vi "sub_calAzimuth.vi"(10 "Index (data block)":i32, 11 "Byte Array":u8[](array[numeric]) format="%x") -> (3 "Azimuth (degree)":dbl format="%#.6f")   [LabVIEW 2020]
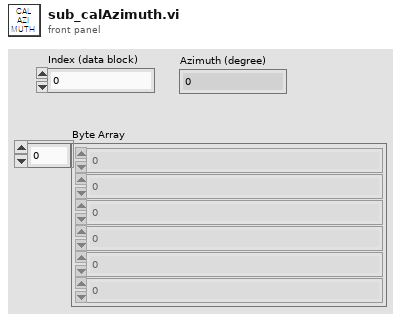
[diagram p1: front panel]
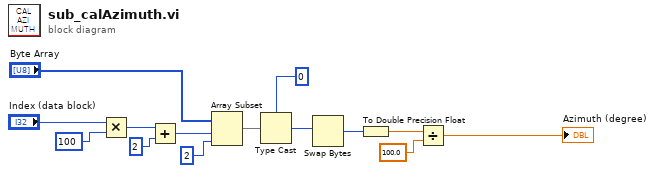
[diagram p0: block diagram]
diagram:
  n1 = Multiply(x="Index (data block)", y=100) -> (x*y=w11:i32)
  n2 = Add(x=w11, y=2) -> (x+y=w9:i32)
  n3 = Array Subset(array="Byte Array", index=w9, length=2 ("길이")) -> (w4:u8[])
  n4 = Type Cast(type=u16 0, x=w4) -> (*(type *) &x=w7:u16)
  n5 = Swap Bytes(anything=w7) -> (byte swapped=w6:u16)
  n6 = To Double Precision Float(number=w6) -> (double precision float=w3:dbl)
  n7 = Divide(x=w3, y=100.0) -> (x/y=→"Azimuth (degree)":dbl)
